vi "General Error Handler MOD.vi"(0 "[error code] (0)":i32 format="%0.0f", 1 "[user-defined codes]":i32[](array[numeric]), 2 "[user-defined descriptions]":string[](array[string]), 5 "[error source] (\" \")":string, 7 "String to Format (not a refnum)":refnum<vi>, 9 "type of dialog (OK msg:1)":T2=enum."OK message", 11 "error in (no error)":errorcluster, 12 "[exception action] (none:0)":i32(ring) items=["no exception", "cancel error on match", "set error on match"], 13 "[exception code]":i32 format="%0.0f", 14 "[exception source]":string) -> (3 "stop event propagated":bool, 4 "STOP?":bool, 10 "message":string=" INSTRUCTIONS:\r\rNormal Use:  When using subVIs that incorporate the error in/error out (or error I/O) structure, place this handler where you want to inform the user of an error, typically at the end of the I/O data path, as the last action of the program.  If the error in error? is ERROR, the handler creates a message describing the error and its source.  If the type of dialog = 1 (default), the message is displayed to the user, who can only acknowledge it.  If the type = 2, the user can acknowledge the message or abort execution; aborting a program with active I/O is not recommended.  If the type = 0, no message is displayed; this is used to process the error programmatically, and the error out cluster elements are wired to individual terminals for that reason.  \r\rOther Use:\n\r\nlocal testing.  To test the error code of a subVI or function that does not have the error I/O structure, you can wire its error code and a source string to the local error code and error source inputs.  If error in error? indicates no error and error code is not equal to 0, the local code and source are substituted for the error in values, and error? is set TRUE (ERROR).", 15 "error out":errorcluster)   [LabVIEW 2012]
doc: "Indicates whether an error occurred. If an error occurred, this VI returns a description of the error and optionally displays a dialog box."
uses:
  <vilib>/Utility/error.llb/DialogTypeEnum.ctl
  <vilib>/Utility/error.llb/whitespace.ctl
panel:
  in  "prompts":T1={"Error %d occurred at %s"="Error %d occurred at %s", "Warning %d occurred at %s"="Warning %d occurred at %s", "Possible reasons: %s"="<b>Possible reason(s):</b>\\n%s", "Error not listed"="This error code is undefined. No one has provided a description for this code, or you might have wired a number that is not an error code to the error code input.", "GetCommError x%lx"="Windows GetCommError:  The hex value of this code is <B>x%04lx</B>.\n\nInterpret it bit-wise as follows:\n<B>x4000</B>: serial port VI error\n<B>x0001</B>: receiving queue overflowed or character was received after end-of-file character\n<B>x0002</B>: character was lost by overwrite\n<B>x0004</B>: parity error\n<B>x0008</B>: framing error\n<B>x0010</B>: break condition\n<B>x0020</B>: CTS timeout\n<B>x0040</B>: DSR timeout\n<B>x0080</B>: RLSD timeout\n<B>x0100</B>: transmission queue was full when new character arrived\n<B>x0200</B>: parallel device timeout\n<B>x0400</B>: parallel device I/O error\n<B>x0800</B>: parallel device not selected\n<B>x1000</B>: parallel device out of paper\n<B>x8000</B>: requested mode is  not supported or the idComDev parameter is invalid.", "Continue"="Continue", "Stop"="Stop", "an unidentified location"="an unidentified location", "No Error"="No Error", "Help"="Why not found?"}
  # "reinitialize to default to display instructions"
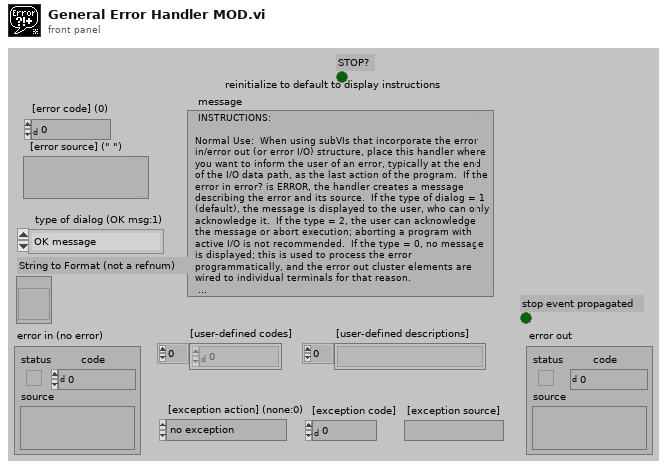
[diagram p1: front panel]
types:
  T1 = cluster{"Error %d occurred at %s":string, "Warning %d occurred at %s":string, "Possible reasons: %s":string, "Error not listed":string, "GetCommError x%lx":string, "Continue":string, "Stop":string, "an unidentified location":string, "No Error":string, "Help":string}
  T2 = typedef "DialogTypeEnum.ctl" = enum16{"no dialog", "OK message", "continue or stop message", "auto error handling dialog", "OK message + warnings", "continue/stop + warnings"}
  T3 = typedef "TagReturnType.ctl" = enum16{"No Tag", "<err>", "<append>"}
  T4 = typedef "whitespace.ctl" = u16
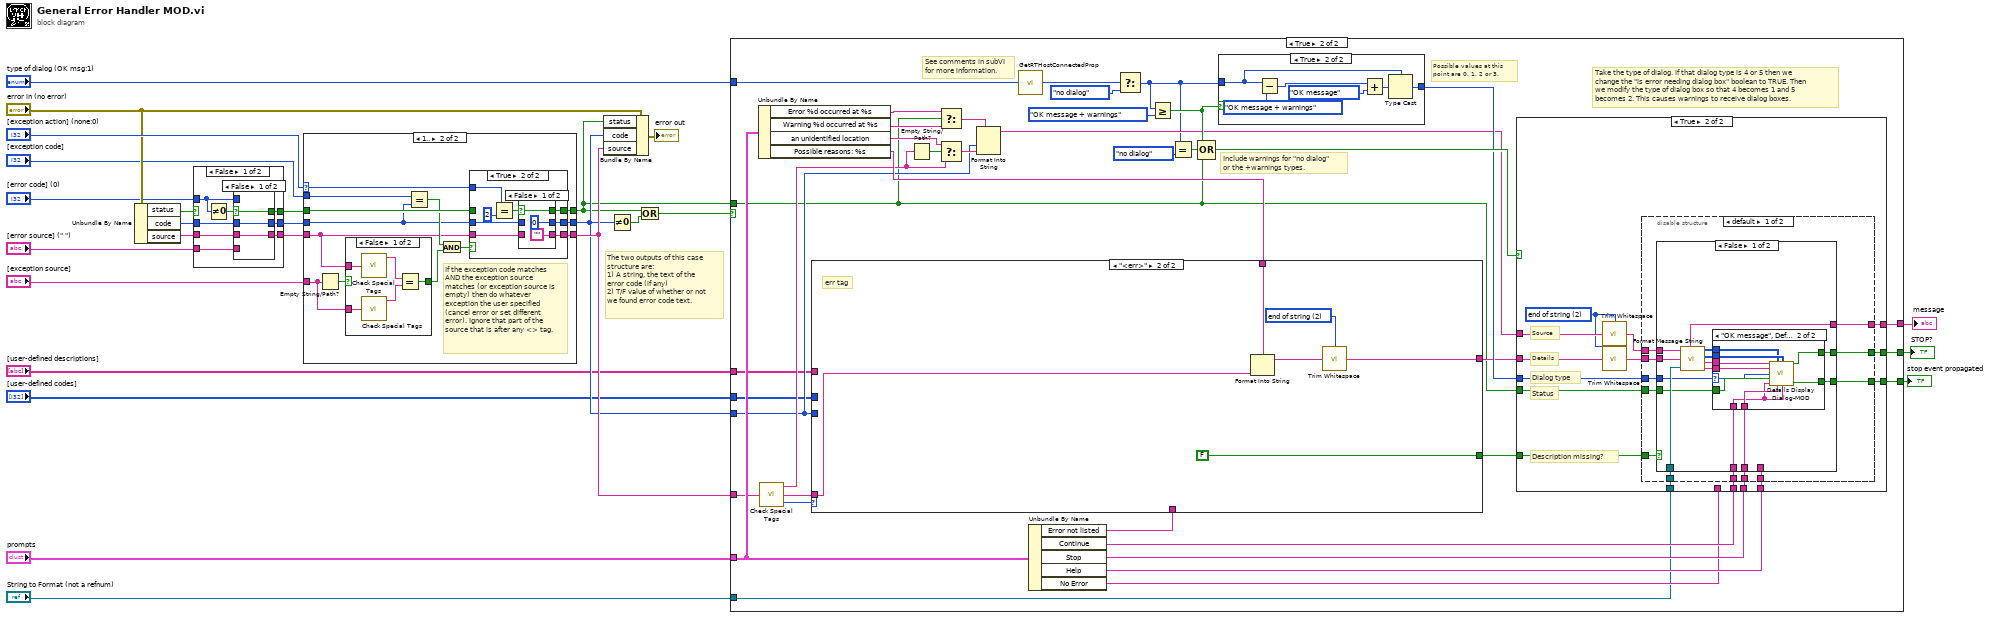
[diagram p0: block diagram]
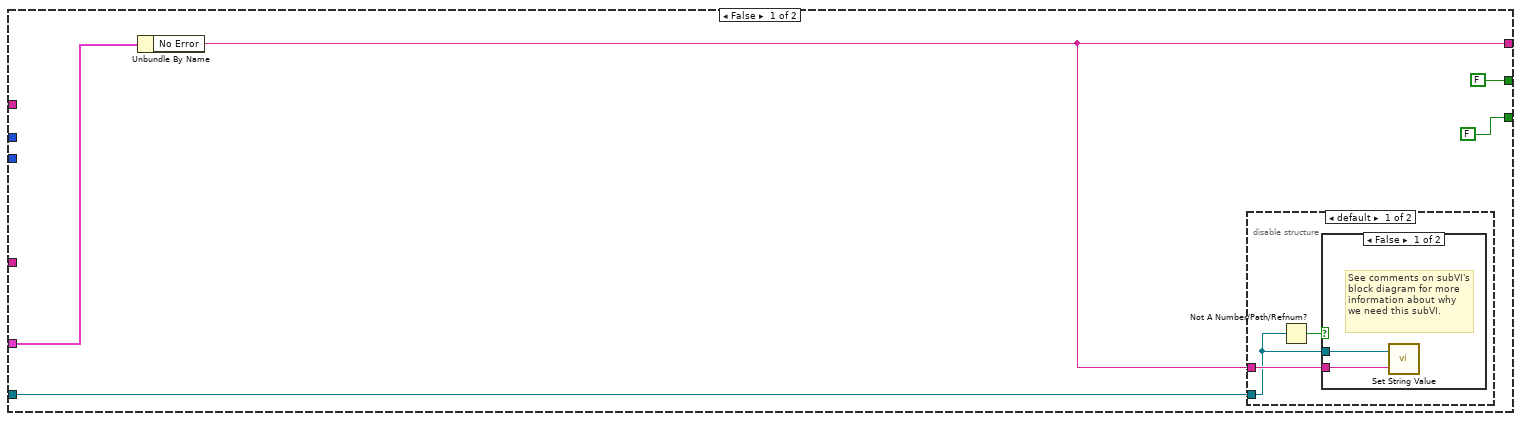
[diagram p8: hidden frame]
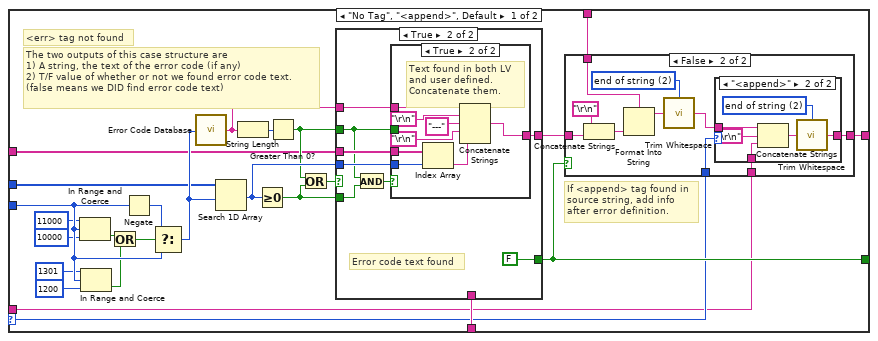
[diagram p12: hidden frame]
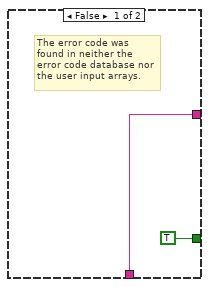
[diagram p15: hidden frame]
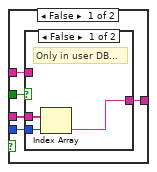
[diagram p16: hidden frame]
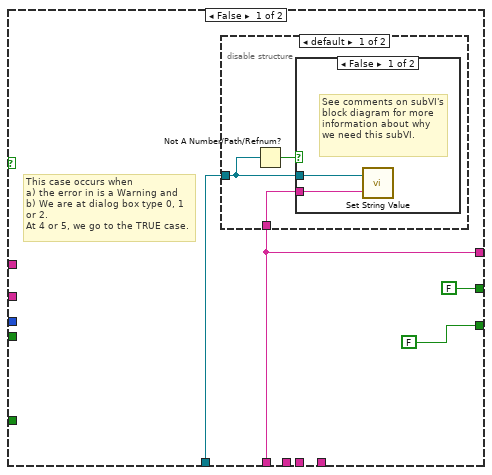
[diagram p18: hidden frame]
diagram:
  # "The two outputs of this case structure are:\n1) A string, the text of the error code (if any)\n2) T/F value of whether or not we found error code text."
  n1 = Unbundle By Name("error in (no error)") -> ("status"=w7:bool, "code"=w21:i32, "source"=w25:string)
  n2 = case shown="False" w7 {
    selector: w7 -> [_ w43]
    tunnel: [w32 w42] -> w23
    tunnel: [w33 w43] -> w22
    tunnel: w21 -> [w29 w42]
    tunnel: [w31 w41] -> w24
    tunnel: w25 -> [w30 w41]
    tunnel: "[error code] (0)" -> [w28 _]
    tunnel: "[error source] (\" \")" -> [w27 _]
    frame False {
      n3 = Not Equal To 0?(x=w28) -> (x != 0?=w34:bool)
      n4 = case shown="False" w34 {
        selector: w34 -> [w37 w40]
        tunnel: [w37 w40] -> w33
        tunnel: w28 -> [_ w39]
        tunnel: [w35 w39] -> w32
        tunnel: w27 -> [_ w38]
        tunnel: [w36 w38] -> w31
        tunnel: w30 -> [w36 _]
        tunnel: w29 -> [w35 _]
        frame False {
        }
        frame True {
        }
      }
    }
    frame True {
    }
  }
  n5 = case shown="1.." "[exception action] (none:0)" {
    selector: "[exception action] (none:0)" -> [_ w51]
    tunnel: [w46 w59] -> w3
    tunnel: w22 -> [w46 w57]
    tunnel: [w45 w58] -> w8
    tunnel: w23 -> [w45 w55]
    tunnel: [w44 w53] -> w18
    tunnel: w24 -> [w44 w49]
    tunnel: "[exception code]" -> [_ w52]
    tunnel: "[exception source]" -> [_ w48]
    frame ..0 {
    }
    frame 1.. {
      # "If the exception code matches AND the exception source matches (or exception source is empty) then do whatever exception the user specified (cancel error or set different error). Ignore that part of the source that is after any <> tag."
      n6 = Empty String/Path?(string/path=w48) -> (empty?=w50:bool)
      n7 = case shown="False" w50 {
        selector: w50 -> [_ w65]
        tunnel: w49 -> [w64 _]
        tunnel: w48 -> [w63 _]
        tunnel: [w62 w65] -> w47
        frame False {
          n8 = call <vilib>:"Check Special Tags.vi"("source"=w64) -> ("Before Tag (source)"=w61:string)  [unwired: 2 out]
          n9 = call <vilib>:"Check Special Tags.vi"("source"=w63) -> ("Before Tag (source)"=w60:string)  [unwired: 2 out]
          n10 = Equal?(x=w61, y=w60) -> (x = y?=w62:bool)
        }
        frame True {
          # "Empty string always matches."
        }
      }
      n11 = Equal?(x=w52, y=w55) -> (x = y?=w56:bool)
      n12 = And(x=w56, y=w47) -> (x .and. y?=w54:bool)
      n13 = case shown="True" w54 {
        tunnel: [w68 w69] -> w59
        tunnel: [w67 w73] -> w58
        tunnel: w57 -> [w68 _]
        tunnel: w55 -> [w67 w72]
        tunnel: w51 -> [_ w76]
        tunnel: [w66 w71] -> w53
        tunnel: w49 -> [w66 w70]
        frame False {
        }
        frame True {
          n14 = Equal?(x=w76, y=2) -> (x = y?=w74:bool)
          n15 = case shown="False" w74 {
            selector: w74 -> [w79 w82]
            tunnel: [0 w81] -> w73
            tunnel: w72 -> [_ w81]
            tunnel: ["" ("Empty String Constant") w80] -> w71
            tunnel: w70 -> [_ w80]
            tunnel: [w79 w82] -> w69
            frame False {
            }
            frame True {
            }
          }
        }
      }
    }
  }
  n16 = Bundle By Name(cluster="error in (no error)", "status"=w3, "code"=w8, "source"=w18) -> (→"error out":errorcluster)
  n17 = Not Equal To 0?(x=w8) -> (x != 0?=w2:bool)
  n18 = Or(x=w3, y=w2) -> (x .or. y?=w19:bool)
  n19 = case shown="True" w19 {
    tunnel: [w85 w112] -> w26
    tunnel: w3 -> [_ w94]
    tunnel: w18 -> [_ w102]
    tunnel: "prompts" -> [w87 w121]
    tunnel: [FALSE ("Stop 2") w115] -> w14
    tunnel: "String to Format (not a refnum)" -> [w84 w108]
    tunnel: w8 -> [_ w100]
    tunnel: "[user-defined descriptions]" -> [_ w98]
    tunnel: "[user-defined codes]" -> [_ w97]
    tunnel: "type of dialog (OK msg:1)" -> [_ w96]
    tunnel: [FALSE ("STOP?") w93] -> w1
    frame False {
      n20 = Unbundle By Name(w87) -> ("No Error"=w85:string)
      n21 = disable-structure shown="default" {
        disable-tunnel: w85 -> [w90 _]
        disable-tunnel: w84 -> [w89 _]
        frame condition #0 (active) {
          n22 = Not A Number/Path/Refnum?(number/path/refnum=w89) -> (NaN/Path/Refnum?=w88:bool)
          n23 = case shown="False" w88 {
            tunnel: w90 -> [w92 _]
            tunnel: w89 -> [w91 _]
            frame False {
              # "See comments on subVI's block diagram for more information about why we need this subVI."
              n24 = call <vilib>:"Set String Value.vi"("No Error"=w92, "String to Format (not a refnum)"=w91) -> ()
            }
            frame True {
            }
          }
        }
        frame condition #1 {
          # "Do nothing in RT case."
        }
      }
    }
    frame True {
      # "See comments in subVI for more information."
      # "Include warnings for \"no dialog\" or the +warnings types."
      # "Possible values at this point are 0, 1, 2 or 3."
      # "Take the type of dialog. If that dialog type is 4 or 5 then we change the \"is error needing dialog box\" boolean to TRUE. Then we modify the type of dialog box so that 4 becomes 1 and 5 becomes 2. This causes warnings to receive dialog boxes."
      n25 = Unbundle By Name(w121) -> ("Error %d occurred at %s"=w99:string, "Warning %d occurred at %s"=w128:string, "an unidentified location"=w125:string, "Possible reasons: %s"=w114:string)
      n26 = call <vilib>:"Check Special Tags.vi"("source"=w102) -> ("Before Tag (source)"=w101:string, "After Tag (special data)"=w129:string, "Tag Found?"=w116:T3)
      n27 = Empty String/Path?(string/path=w101) -> (empty?=w130:bool)
      n28 = Select(t=w99, s=w94, f=w128) -> (s? t:f=w127:string)
      n29 = Select(t=w125, s=w130, f=w101) -> (s? t:f=w126:string)
      n30 = Format Into String(format string=w127, w100, w126) -> (resulting string=w110:string)  [unwired: 2 in, 1 out]
      n31 = call <vilib>:"GetRTHostConnectedProp.vi"() -> ("App.RTHostConnected"=w95:bool)
      n32 = Unbundle By Name(w121) -> ("Error not listed"=w124:string, "Continue"=w123:string, "Stop"=w122:string, "Help"=w119:string, "No Error"=w109:string)
      n33 = case shown="\"<err>\"" w116 {
        selector: w116 -> [w143 _]
        tunnel: [w141 w211] -> w111
        tunnel: w100 -> [w162 _]
        tunnel: w129 -> [w142 w210]
        tunnel: w124 -> [w161 _]
        tunnel: [w144 FALSE] -> w120
        tunnel: w114 -> [w146 w209]
        tunnel: w98 -> [w139 _]
        tunnel: w97 -> [w138 _]
        frame "No Tag", "<append>", Default {
          # "If <append> tag found in source string, add info after error definition."
          # "<err> tag not found"
          # "The two outputs of this case structure are\n1) A string, the text of the error code (if any)\n2) T/F value of whether or not we found error code text.\n(false means we DID find error code text)"
          n34 = In Range and Coerce(upper limit=11000, x=w162, lower limit=10000) -> (In Range?=w154:bool)  [unwired: 1 out]
          n35 = In Range and Coerce(upper limit=1301, x=w162, lower limit=1200) -> (In Range?=w155:bool)  [unwired: 1 out]
          n36 = Or(x=w154, y=w155) -> (x .or. y?=w153:bool)
          n37 = Negate(x=w162) -> (-x=w157:i32)
          n38 = Select(t=w157, s=w153, f=w162) -> (s? t:f=w140:i32)
          n39 = call <vilib>:"Error Code Database.vi"("Error Code"=w140) -> ("Error Text"=w147:string)
          n40 = Search 1D Array(1D array=w138, element=w140) -> (index of element=w160:i32)  [unwired: 1 out]
          n41 = String Length(string=w147) -> (length=w151:i32)
          n42 = Greater Or Equal To 0?(x=w160) -> (x >= 0?=w148:bool)
          n43 = Greater Than 0?(x=w151) -> (x > 0?=w149:bool)
          n44 = Or(x=w149, y=w148) -> (x .or. y?=w150:bool)
          n45 = case shown="True" w150 {
            tunnel: w160 -> [_ w186]
            tunnel: [w182 w184] -> w145
            tunnel: w161 -> [w182 _]
            tunnel: [TRUE FALSE] -> w144
            tunnel: w149 -> [_ w183]
            tunnel: w148 -> [_ w188]
            tunnel: w139 -> [_ w187]
            tunnel: w147 -> [_ w185]
            frame False {
              # "The error code was found in neither the error code database nor the user input arrays."
            }
            frame True {
              # "Error code text found"
              n46 = And(x=w183, y=w188) -> (x .and. y?=w189:bool)
              n47 = case shown="True" w189 {
                tunnel: w187 -> [w192 w207]
                tunnel: w186 -> [w191 w206]
                tunnel: w185 -> [w193 w200]
                tunnel: [w194 w204] -> w184
                tunnel: w183 -> [w195 _]
                frame False {
                  n48 = case shown="False" w195 {
                    tunnel: [w196 w199] -> w194
                    tunnel: w193 -> [_ w199]
                    tunnel: w192 -> [w198 _]
                    tunnel: w191 -> [w197 _]
                    frame False {
                      # "Only in user DB..."
                      n49 = Index Array(array=w198, index=w197) -> (element=w196:string)
                    }
                    frame True {
                      # "Only in LV DB..."
                    }
                  }
                }
                frame True {
                  # "Text found in both LV\nand user defined. \nConcatenate them."
                  n50 = Index Array(array=w207, index=w206) -> (element=w205:string)
                  n51 = Concatenate Strings(w200, "\r\n" ("End of Line Constant"), "---" ("string"), "\r\n" ("End of Line Constant"), w205) -> (w204:string)
                }
              }
            }
          }
          n52 = case shown="False" w144 {
            tunnel: w146 -> [_ w173]
            tunnel: [w163 w165] -> w141
            tunnel: w145 -> [w163 w170]
            tunnel: w143 -> [_ w167]
            tunnel: w142 -> [_ w166]
            frame True {
              # "no explanation given for error."
            }
            frame False {
              w164 = T4 2 items=["both", "start of string", "end of string"] ("location (both)")
              n53 = Concatenate Strings("\r\n" ("End of Line Constant"), w170) -> (w171:string)
              n54 = Format Into String(format string=w173, w171) -> (resulting string=w172:string)  [unwired: 2 in, 1 out]
              n55 = call <vilib>:"Trim Whitespace.vi"("string"=w172, "location (both)"=w164) -> ("trimmed string"=w168:string)
              n56 = case shown="\"<append>\"" w167 {
                tunnel: w168 -> [w174 w179]
                tunnel: [w174 w176] -> w165
                tunnel: w166 -> [_ w178]
                frame "No Tag", Default {
                }
                frame "<append>" {
                  w175 = T4 2 items=["both", "start of string", "end of string"] ("location (both)")
                  n57 = Concatenate Strings(w179, "\r\n" ("End of Line Constant"), w178) -> (w177:string)
                  n58 = call <vilib>:"Trim Whitespace.vi"("string"=w177, "location (both)"=w175) -> ("trimmed string"=w176:string)
                }
              }
            }
          }
        }
        frame "<err>" {
          w208 = T4 2 items=["both", "start of string", "end of string"] ("location (both)")
          # "err tag"
          n59 = Format Into String(format string=w209, w210) -> (resulting string=w212:string)  [unwired: 2 in, 1 out]
          n60 = call <vilib>:"Trim Whitespace.vi"("string"=w212, "location (both)"=w208) -> ("trimmed string"=w211:string)
        }
      }
      n61 = Select(t=w96, s=w95, f=DialogTypeEnum."no dialog" ("type of dialog (OK msg:1)")) -> (s? t:f=w103:T2)
      n62 = Greater Or Equal?(x=w103, y=DialogTypeEnum."OK message + warnings" ("type of dialog (OK msg:1)")) -> (x >= y?=w117:bool)
      n63 = Equal?(x=w103, y=DialogTypeEnum."no dialog" ("type of dialog (OK msg:1)")) -> (x = y?=w107:bool)
      n64 = Compound Arithmetic op=OR(w117, w107, w94) -> (w118:bool)
      n65 = case shown="True" w117 {
        tunnel: w103 -> [w131 w132]
        tunnel: [w131 w134] -> w113
        frame False {
        }
        frame True {
          n66 = Subtract(x=w132, y=DialogTypeEnum."OK message + warnings" ("type of dialog (OK msg:1)")) -> (x-y=w137:u16)
          n67 = Add(x=w137, y=DialogTypeEnum."OK message" ("type of dialog (OK msg:1)")) -> (x+y=w133:u16)
          n68 = Type Cast(type=w132, x=w133) -> (*(type *) &x=w134:T2)
        }
      }
      n69 = case shown="True" w118 {
        tunnel: w113 -> [_ w237]
        tunnel: w123 -> [_ w236]
        tunnel: w122 -> [_ w235]
        tunnel: w120 -> [_ w224]
        tunnel: w119 -> [_ w234]
        tunnel: w110 -> [_ w227]
        tunnel: w111 -> [_ w228]
        tunnel: w94 -> [_ w233]
        tunnel: [FALSE ("Stop 2") w232] -> w115
        tunnel: [w215 w231] -> w112
        tunnel: w109 -> [w215 _]
        tunnel: w108 -> [w216 w230]
        tunnel: [FALSE ("STOP?") w223] -> w93
        frame False {
          # "This case occurs when\na) the error in is a Warning and\nb) We are at dialog box type 0, 1 or 2.\nAt 4 or 5, we go to the TRUE case."
          n70 = disable-structure shown="default" {
            disable-tunnel: w216 -> [w220 _]
            disable-tunnel: w215 -> [w218 _]
            frame condition #0 (active) {
              n71 = Not A Number/Path/Refnum?(number/path/refnum=w220) -> (NaN/Path/Refnum?=w219:bool)
              n72 = case shown="False" w219 {
                tunnel: w218 -> [w222 _]
                tunnel: w220 -> [w221 _]
                frame False {
                  # "See comments on subVI's block diagram for more information about why we need this subVI."
                  n73 = call <vilib>:"Set String Value.vi"("No Error"=w222, "String to Format (not a refnum)"=w221) -> ()
                }
                frame True {
                }
              }
            }
            frame condition #1 {
              # "Do nothing in RT case."
            }
          }
        }
        frame True {
          w225 = T4 2 items=["both", "start of string", "end of string"] ("location (both)")
          # "Description missing?"
          # "Dialog type"
          # "Status"
          # "Details"
          # "Source"
          n74 = call <vilib>:"Trim Whitespace.vi"("string"=w227, "location (both)"=w225) -> ("trimmed string"=w226:string)
          n75 = call <vilib>:"Trim Whitespace.vi"("string"=w228, "location (both)"=w225) -> ("trimmed string"=w229:string)
          n76 = disable-structure "Conditional Disable Structure" shown="default" {
            disable-tunnel: w237 -> [w249 w297]
            disable-tunnel: w236 -> [w248 w296]
            disable-tunnel: w235 -> [w247 w295]
            disable-tunnel: w234 -> [w246 _]
            disable-tunnel: w233 -> [w245 _]
            disable-tunnel: [w244 w294] -> w232
            disable-tunnel: [w243 w293] -> w231
            disable-tunnel: w230 -> [w242 w292]
            disable-tunnel: w229 -> [w241 w291]
            disable-tunnel: w226 -> [w240 w290]
            disable-tunnel: w224 -> [w239 _]
            disable-tunnel: [w238 _] -> w223
            frame condition #0 (active) {
              n77 = case shown="False" w239 {
                tunnel: w241 -> [w262 w281]
                tunnel: w246 -> [_ w287]
                tunnel: w248 -> [w258 w285]
                tunnel: w247 -> [w257 w284]
                tunnel: w249 -> [w260 w286]
                tunnel: [w259 w283] -> w244
                tunnel: w240 -> [w263 w282]
                tunnel: w245 -> [w256 _]
                tunnel: [w251 w279] -> w243
                tunnel: w242 -> [w261 w277]
                tunnel: [w250 FALSE ("STOP?")] -> w238
                frame False {
                  n78 = call <vilib>:"Format Message String.vi"("Source"=w263, "Details"=w262, "String to Format (not a refnum)"=w261) -> ("message"=w251:string, "Bold Start"=w255:i32[], "Bold Length"=w254:i32[], "Source Out"=w253:string, "Details Out"=w252:string)  [unwired: 1 out]
                  n79 = case shown="\"OK message\", Default" w260 {
                    selector: w260 -> [_ w269]
                    tunnel: [FALSE ("stop event propagated") w275] -> w259
                    tunnel: w258 -> [_ w271]
                    tunnel: w257 -> [_ w272]
                    tunnel: w256 -> [_ w270]
                    tunnel: w255 -> [_ w273]
                    tunnel: w254 -> [_ w274]
                    tunnel: w253 -> [_ w267]
                    tunnel: w252 -> [_ w268]
                    tunnel: [FALSE ("STOP?") w266] -> w250
                    frame "no dialog" {
                    }
                    frame "OK message", Default {
                      n80 = call "Details Display Dialog-MOD.vi"("Source"=w267, "Start"=w273, "Length"=w274, "Details"=w268, "dialog type"=w269, "Error or Warning"=w270, "contname"=w271, "stopname"=w272, "okname"=w271) -> ("STOP?"=w266:bool, "stop event propagated"=w275:bool)  [unwired: 5 out]
                    }
                  }
                }
                frame True {
                  w280 = "\r\n" ("End of Line Constant")
                  n81 = Concatenate Strings(w282, w280, w280, w281) -> (w279:string)
                  n82 = Not A Number/Path/Refnum?(number/path/refnum=w277) -> (NaN/Path/Refnum?=w278:bool)
                  n83 = call <vilib>:"Not Found Dialog.vi"("Help"=w287, "Message"=w279, "Stop"=w284, "Continue"=w285, "type of dialog (OK msg:1)"=w286) -> ("stop event propagated"=w283:bool)  [unwired: 1 in]
                  n84 = case shown="False" w278 {
                    tunnel: w277 -> [w289 _]
                    tunnel: w279 -> [w288 _]
                    frame False {
                      n85 = call <vilib>:"Set String Value.vi"("No Error"=w288, "String to Format (not a refnum)"=w289) -> ()
                    }
                    frame True {
                    }
                  }
                }
              }
            }
            frame condition #1 {
              n86 = call <vilib>:"Format Message String.vi"("Source"=w290, "Details"=w291, "String to Format (not a refnum)"=w292) -> ("message"=w293:string)  [unwired: 1 in, 4 out]
              n87 = case shown="\"continue or stop message\", \"continue/stop + warnings\"" w297 {
                tunnel: [FALSE ("stop event propagated") FALSE ("stop event propagated") FALSE ("stop event propagated") w308] -> w294
                tunnel: w293 -> [_ w300 w307 w312]
                tunnel: w296 -> [_ w299 w306 w311]
                tunnel: w295 -> [_ _ w305 w310]
                frame "no dialog" {
                }
                frame "OK message", "OK message + warnings", Default {
                  n88 = One Button Dialog(message=w300, button name ("OK")=w299) -> ()  [unwired: 1 out]
                }
                frame "continue or stop message", "continue/stop + warnings" {
                  n89 = Two Button Dialog(message=w307, 1:w305, 2:w306) -> (T button?=w303:bool)
                  n90 = Not(x=w303) -> (.not. x?=w302:bool)
                  n91 = Stop(stop? (T)=w302) -> ()
                }
                frame "auto error handling dialog" {
                  n92 = Two Button Dialog(message=w312, 1:w310, 2:w311) -> (T button?=w309:bool)
                  n93 = Not(x=w309) -> (.not. x?=w308:bool)
                }
              }
            }
          }
        }
      }
    }
  }
  "message" <- w26
  "stop event propagated" <- w14
  "STOP?" <- w1
